vi "PhaseCalculationCount.vi"(11 "Phase":dbl) -> (3 "PhaseCount":u64)   [LabVIEW 2018]
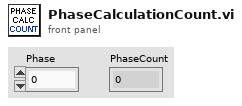
[diagram p1: front panel]
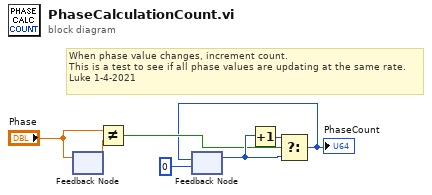
[diagram p0: block diagram]
diagram:
  # "When phase value changes, increment count.\nThis is a test to see if all phase values are updating at the same rate.\nLuke 1-4-2021"
  n1 = feedback #1() -> (w3:dbl)  [unwired: 1 in]
  n2 = feedback-in #1("Phase") -> ()
  n3 = Not Equal?(x="Phase", y=w3) -> (x != y?=w5:bool)
  n4 = feedback #2(u64 0) -> (w7:u64)
  n5 = Increment(x=w7) -> (x+1=w6:u64)
  n6 = Select(t=w6, s=w5, f=w7) -> (s? t:f=w1:u64)
  "PhaseCount" <- w1
  n7 = feedback-in #2(w1) -> ()
